vi "_main_SM_tdms.vi"(8 "error in":errorcluster, 10 "Variant":variant, 11 "Enum":T1) -> (0 "error out":errorcluster)   [LabVIEW 2023]
uses:
  ctl_tdms.ctl
  ctl_structure_type.ctl
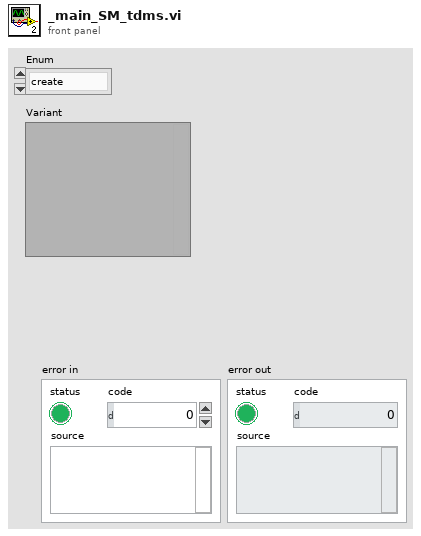
[diagram p1: front panel]
types:
  T1 = typedef "ctl_tdms.ctl" = enum16{"create", "write_text", "write_data", "close"}
  T2 = enum16{"open", "open or create", "create or replace", "create", "open (read-only)"}
  T3 = typedef "ctl_structure_type.ctl" = cluster{"group":string, "channel_name":string, "channel data":dbl[], "channel STRING":string, "Properties names":string[], "Properties values":string[]}
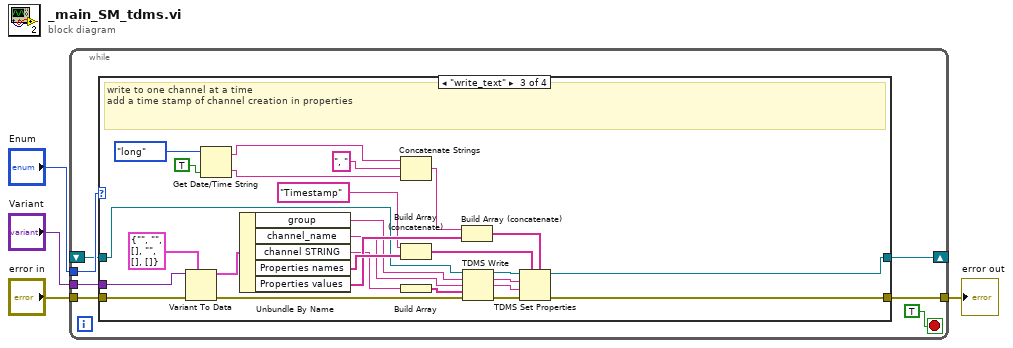
[diagram p0: block diagram]
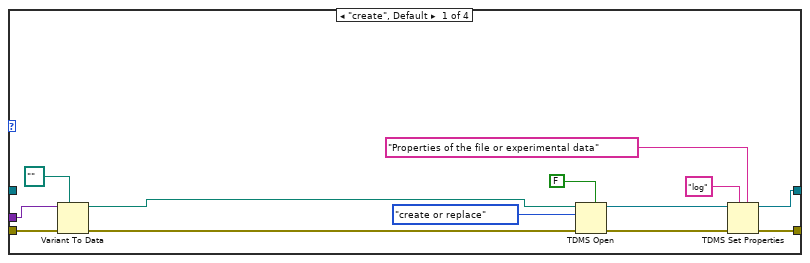
[diagram p2: hidden frame]
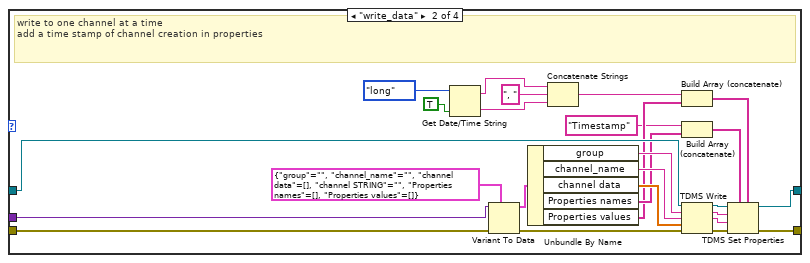
[diagram p3: hidden frame]
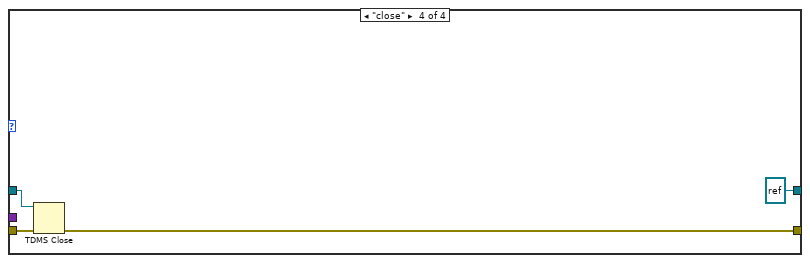
[diagram p4: hidden frame]
diagram:
  n1 = while {
    tunnel: "Enum" -> [w10]
    tunnel: "Variant" -> [w9]
    tunnel: "error in" -> [w8]
    tunnel: [w7] -> w1
    shift-right: [w6] -> _
    shift-left: _ -> [w5]
    stop <- TRUE stop-if-true
    n2 = case shown="\"write_text\"" w10 {
      tunnel: w9 -> [w24 w45 w73 _]
      tunnel: w8 -> [w23 w49 w77 w78]
      tunnel: [w16 w39 w69 w81] -> w7
      tunnel: [w14 w40 w70 refnum<k34> refnum ("tdms file out")] -> w6
      tunnel: w5 -> [_ w50 w55 w79]
      frame "create", Default {
        n3 = Variant To Data(error in=w23, type=path "" ("path"), Variant=w24) -> (data=w21:path, error out=w19:errorcluster)
        n4 = TDMS Open(5:FALSE ("create index file? (T)"), 8:w19, 10:T2."create or replace" ("operation (0:open)"), 11:w21) -> (0:w17:errorcluster, 3:w15:refnum<k34>)  [unwired: 3 in]
        n5 = TDMS Set Properties(5:"Properties of the file or experimental data", 7:"log", 8:w17, 11:w15) -> (0:w16:errorcluster, 3:w14:refnum<k34>)  [unwired: 2 in, 2 out]
      }
      frame "write_data" {
        # "write to one channel at a time\nadd a time stamp of channel creation in properties"
        n6 = Get Date/Time String(date format (0)=enum16{"short", "long", "abbreviated"}."long", want seconds? (F)=TRUE) -> (date string=w29:string, time string=w28:string)  [unwired: 1 in]
        n7 = Variant To Data(error in=w49, type=T3 {"group"="", "channel_name"="", "channel data"=[], "channel STRING"="", "Properties names"=[], "Properties values"=[]}, Variant=w45) -> (data=w47:T3, error out=w48:errorcluster)
        n8 = Unbundle By Name(w47) -> ("group"=w44:string, "channel_name"=w36:string, "channel data"=w43:dbl[], "Properties names"=w35:string[], "Properties values"=w33:string[])
        n9 = Concatenate Strings(w29, ", " ("string"), w28) -> (w26:string)
        n10 = Build Array (concatenate)(w26, w33) -> (w32:string[])
        n11 = Build Array (concatenate)("Timestamp" ("string"), w35) -> (w34:string[])
        n12 = TDMS Write(0:w50, 5:w44, 7:w36, 9:w43, 11:w48) -> (4:w41:refnum<k34>, 6:w37:string, 8:w38:string, 15:w42:errorcluster)  [unwired: 1 in]
        n13 = TDMS Set Properties(5:w32, 7:w34, 8:w42, 9:w38, 10:w37, 11:w41) -> (0:w39:errorcluster, 3:w40:refnum<k34>)  [unwired: 2 out]
      }
      frame "write_text" {
        # "write to one channel at a time\nadd a time stamp of channel creation in properties"
        n14 = Variant To Data(error in=w77, type=T3 {"group"="", "channel_name"="", "channel data"=[], "channel STRING"="", "Properties names"=[], "Properties values"=[]}, Variant=w73) -> (data=w75:T3, error out=w76:errorcluster)
        n15 = Get Date/Time String(date format (0)=enum16{"short", "long", "abbreviated"}."long", want seconds? (F)=TRUE) -> (date string=w60:string, time string=w59:string)  [unwired: 1 in]
        n16 = Unbundle By Name(w75) -> ("group"=w52:string, "channel_name"=w51:string, "channel STRING"=w54:string, "Properties names"=w66:string[], "Properties values"=w64:string[])
        n17 = Concatenate Strings(w60, ", " ("string"), w59) -> (w57:string)
        n18 = Build Array (concatenate)("Timestamp" ("string"), w66) -> (w65:string[])
        n19 = Build Array(w54) -> (w53:string[])
        n20 = Build Array (concatenate)(w57, w64) -> (w63:string[])
        n21 = TDMS Write(0:w55, 5:w52, 7:w51, 9:w53, 11:w76) -> (4:w71:refnum<k34>, 6:w67:string, 8:w68:string, 15:w72:errorcluster)  [unwired: 1 in]
        n22 = TDMS Set Properties(5:w63, 7:w65, 8:w72, 9:w68, 10:w67, 11:w71) -> (0:w69:errorcluster, 3:w70:refnum<k34>)  [unwired: 2 out]
      }
      frame "close" {
        n23 = TDMS Close(8:w78, 11:w79) -> (0:w81:errorcluster)  [unwired: 1 out]
      }
    }
  }
  "error out" <- w1
